vi "Read Analogue.vi"(8 "error in (no error)":errorcluster, 11 "HiPOT Instrument":refnum<class "HiPOT Instrument.lvclass">) -> (0 "error out":errorcluster, 2 "Waveforms":waveform(dbl)[](array[waveform]), 3 "HiPOT Instrument out":refnum<class "HiPOT Instrument.lvclass">)   [LabVIEW 2025, in "HiPOT.lvlib" / "HiPOT Instrument.lvclass"]
uses:
  HiPOT Instrument.lvclass
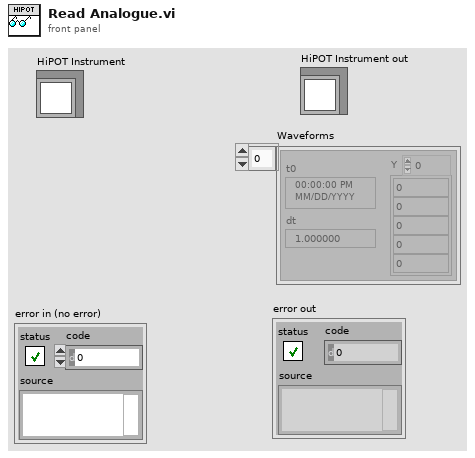
[diagram p1: front panel]
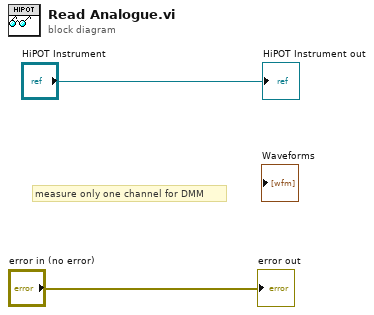
[diagram p0: block diagram]
diagram:
  # "measure only one channel for DMM"
  "error out" <- "error in (no error)"
  "HiPOT Instrument out" <- "HiPOT Instrument"
